vi "Reports.Results JSON V1 to JSON V2 File.vi"(8 "error in (no error)":errorcluster, 9 "JSONV1 Data File":path, 10 "File Name":string, 11 "Output Folder":path) -> (0 "error out":errorcluster)   [LabVIEW 2018]
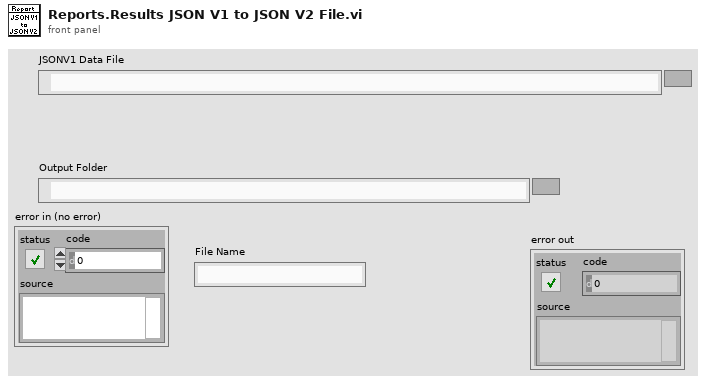
[diagram p1: front panel]
types:
  T1 = typedef "Report.Result Data JSON V2.0.0.ctl" = cluster{"Type":string, "Version":string, "TestEvent":T2, "UUTInfo":T4, "Station":T5, "TestSequence":T6, "NumericData":T7[], "AttributeData":T8[], "DataObjs":T9[]}
  T2 = typedef "Report.Result Test Event.ctl" = cluster{"ProcessStep":string, "StartTime":string, "EndTime":string, "Mode":string, "Operator":string, "Comment":string, "Result":T3}
  T3 = typedef "Report.Result State.ctl" = cluster{"State":string, "Code":i32, "Desc":string, "Details":string}
  T4 = typedef "Report.Result UUTInfo.ctl" = cluster{"PN":string, "SN":string, "LotNumber":string, "DateCode":string, "AltID":string, "Properties":cluster{"Name":string, "Value":string}[], "Revision":string}
  T5 = typedef "Report.Result Test Station.ctl" = cluster{"Name":string, "Location":string, "ConfigID":string, "PCName":string, "Slot":string}
  T6 = typedef "Report.Result Test Sequence.ctl" = cluster{"Name":string, "Setup":cluster{"Name":string, "Value":string}[]}
  T7 = typedef "Report.Result Numeric.ctl" = cluster{"Cnt":i32, "Step":string, "Category":string, "Name":string, "Value":dbl, "Units":string, "LimType":string, "LL":dbl, "UL":dbl, "Time":string, "Result":T3}
  T8 = typedef "Report.Result Attribute.ctl" = cluster{"Cnt":i32, "Step":string, "Category":string, "Name":string, "Value":string, "Units":string, "LimType":string, "LL":string, "UL":string, "Time":string, "Result":T3}
  T9 = typedef "Report.Result DataObject.ctl" = cluster{"Cnt":i32, "Step":string, "Category":string, "Name":string, "Type":string, "File Name":string, "Time":string}
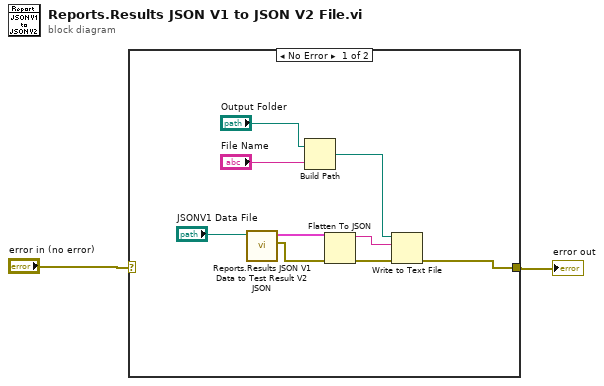
[diagram p0: block diagram]
diagram:
  n1 = case shown="No Error" "error in (no error)" {
    selector: "error in (no error)" -> [_ w12]
    tunnel: [w3 w12] -> w1
    frame No Error {
      n2 = call "Reports.Results JSON V1 Data to Test Result V2 JSON.vi"("JSON V1File"="JSONV1 Data File") -> ("error out"=w4:errorcluster, "Test Result V2"=w10:T1)  [unwired: 7 in]
      n3 = Build Path(base path="Output Folder", name or relative path="File Name") -> (appended path=w8:path)
      n4 = Flatten To JSON(anything=w10, error in (no error)=w4) -> (JSON string=w11:string, 11:w9:errorcluster)  [unwired: 1 in]
      n5 = Write to Text File(file (use dialog)=w8, text=w11, error in=w9) -> (error out=w3:errorcluster)  [unwired: 1 in, 2 out]
    }
    frame Error {
    }
  }
  "error out" <- w1
